vi "logic-train-sample-7-1-ALT.vi"(11 "Request\nCapture":bool) -> (1 "Hand_Close":bool, 3 "Arm_Extend":bool, 4 "State":T1)   [LabVIEW 2020]
uses:
  sample-7-1-state-enum.ctl
  <vilib>/Utility/semaphor.llb/Obtain Semaphore Reference.vi
  <vilib>/Rock Robotics/WPI/ThirdParty/JAS_Junk/TrajLib/Timer_Reset.vi
  <vilib>/Rock Robotics/WPI/ThirdParty/JAS_Junk/TrajLib/Timer_Start.vi
  <vilib>/Rock Robotics/WPI/ThirdParty/JAS_Junk/TrajLib/Timer_Stop.vi
  <vilib>/Rock Robotics/WPI/ThirdParty/JAS_Junk/TrajLib/Trajectory_Library.lvlib
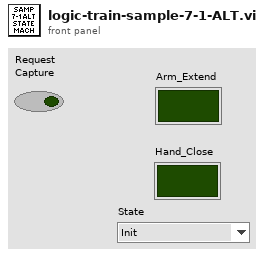
[diagram p1: front panel]
types:
  T1 = typedef "sample-7-1-state-enum.ctl" = enum16{"Init", "ExtendArm", "ExtendArmWait", "CloseHand", "CloseHandWait", "RetractArm", "RetractArmWait", "OpenHand", "OpenHandWait", "Ready"}
  T2 = typedef "Trajectory_Library.lvlib/TIMER.ctl" = cluster{"StartTime":dbl, "Accumulated TIme":dbl, "Running":bool, "semaphore":T3}
  T3 = typedef "Semaphore RefNum" = refnum<k1>
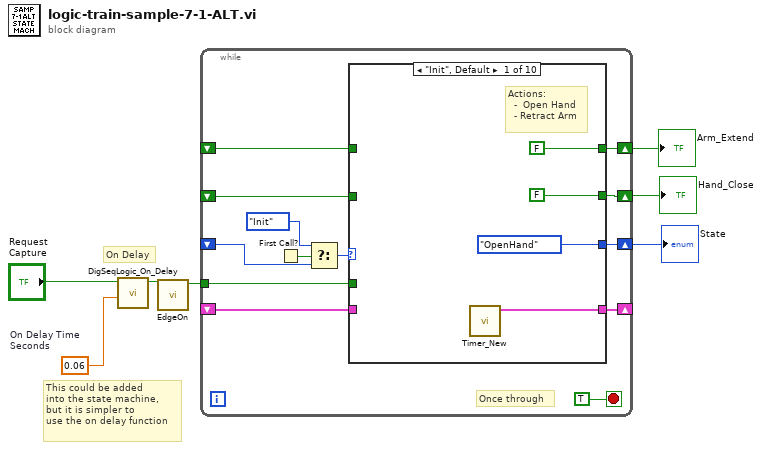
[diagram p0: block diagram]
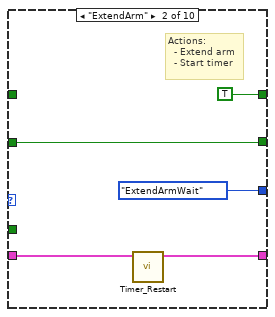
[diagram p2: hidden frame]
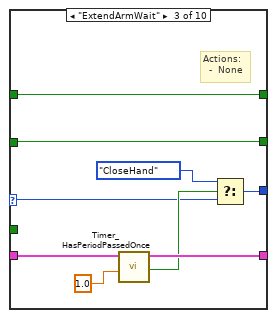
[diagram p3: hidden frame]
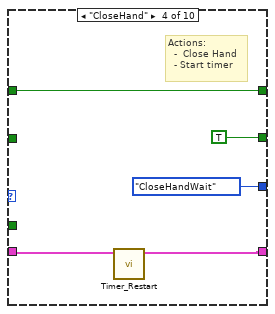
[diagram p4: hidden frame]
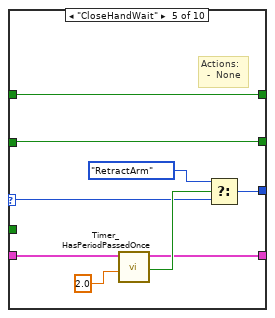
[diagram p5: hidden frame]
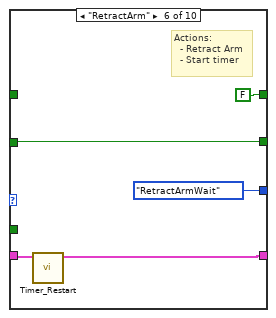
[diagram p6: hidden frame]
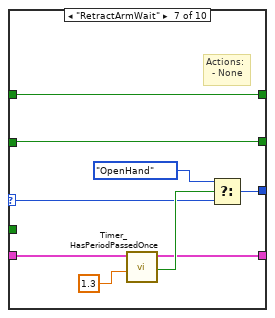
[diagram p7: hidden frame]
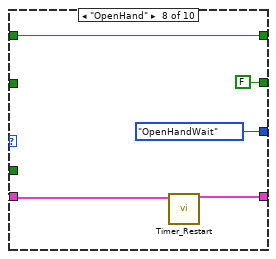
[diagram p8: hidden frame]
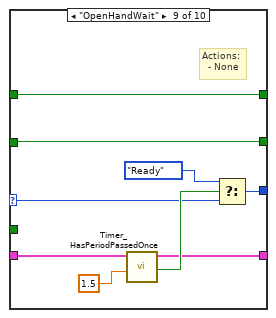
[diagram p9: hidden frame]
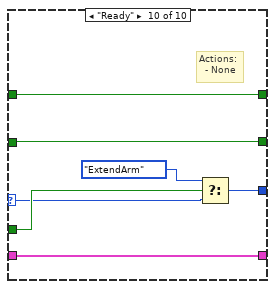
[diagram p10: hidden frame]
diagram:
  w7 = 0.06  # On Delay Time Seconds
  # "This could be added\ninto the state machine,\nbut it is simpler to \nuse the on delay function"
  # "On Delay"
  n1 = call <vilib>:"DigSeqLogic_On_Delay.vi"("Delay"=w7, "Input"="Request\nCapture") -> ("Output"=w6:bool)  [unwired: 8 in, 1 out]
  n2 = call "EdgeOn.vi"("Input"=w6) -> ("Edge On"=w4:bool)  [unwired: 10 in]
  n3 = while {
    shift-right: [w13] -> w1
    shift-left: _ -> [w16]
    shift-right: [w14] -> w2
    shift-left: _ -> [w19]
    shift-right: [w15] -> w3
    shift-left: _ -> [w10]
    shift-right: [w12] -> _
    shift-left: _ -> [w20]
    tunnel: w4 -> [w18]
    stop <- TRUE stop-if-true
    # "Once through"
    n4 = First Call?() -> (First Call?: T/F=w9:bool)
    n5 = Select(t=sample-7-1-state-enum."Init" ("Sample-7-1-State"), s=w9, f=w10) -> (s? t:f=w11:T1)
    n6 = case shown="\"Init\", Default" w11 {
      selector: w11 -> [_ _ w30 _ w48 _ w63 _ w76 w83]
      tunnel: [FALSE TRUE w37 w43 w44 FALSE w59 w68 w72 w87] -> w13
      tunnel: [FALSE w28 w38 TRUE w45 w54 w58 FALSE w73 w86] -> w14
      tunnel: [sample-7-1-state-enum."OpenHand" ("Sample-7-1-State") sample-7-1-state-enum."ExtendArmWait" ("Sample-7-1-State") w32 sample-7-1-state-enum."CloseHandWait" ("Sample-7-1-State") w49 sample-7-1-state-enum."RetractArmWait" ("Sample-7-1-State") w62 sample-7-1-state-enum."OpenHandWait" ("Sample-7-1-State") w77 w81] -> w15
      tunnel: [w21 w25 w35 w42 w46 w57 w60 w70 w74 w85] -> w12
      tunnel: w20 -> [_ w26 w34 w41 w47 w53 w61 w69 w75 w85]
      tunnel: w19 -> [_ w28 w38 _ w45 w54 w58 _ w73 w86]
      tunnel: w16 -> [_ _ w37 w43 w44 _ w59 w68 w72 w87]
      tunnel: w18 -> [_ _ _ _ _ _ _ _ _ w84]
      frame "Init", Default {
        # "Actions:\n  -  Open Hand\n  - Retract Arm"
        n7 = call <vilib>:"Timer_New.vi"() -> ("TIMER"=w21:T2)  [unwired: 11 in]
      }
      frame "ExtendArm" {
        # "Actions:\n  - Extend arm\n  - Start timer"
        n8 = call <vilib>:"Timer_Restart.vi"("in Timer"=w26) -> ("out Timer"=w25:T2)  [unwired: 10 in]
      }
      frame "ExtendArmWait" {
        # "Actions:\n  -  None"
        n9 = call <vilib>:"Timer_HasPeriodPassedOnce.vi"("Period"=1.0, "in Timer"=w34) -> ("Expired"=w31:bool, "out Timer"=w35:T2)  [unwired: 7 in, 1 out]
        n10 = Select(t=sample-7-1-state-enum."CloseHand" ("Sample-7-1-State"), s=w31, f=w30) -> (s? t:f=w32:T1)
      }
      frame "CloseHand" {
        # "Actions:\n  -  Close Hand\n  - Start timer"
        n11 = call <vilib>:"Timer_Restart.vi"("in Timer"=w41) -> ("out Timer"=w42:T2)  [unwired: 10 in]
      }
      frame "CloseHandWait" {
        # "Actions:\n  -  None"
        n12 = call <vilib>:"Timer_HasPeriodPassedOnce.vi"("Period"=2.0, "in Timer"=w47) -> ("Expired"=w50:bool, "out Timer"=w46:T2)  [unwired: 7 in, 1 out]
        n13 = Select(t=sample-7-1-state-enum."RetractArm" ("Sample-7-1-State"), s=w50, f=w48) -> (s? t:f=w49:T1)
      }
      frame "RetractArm" {
        # "Actions:\n  - Retract Arm\n  - Start timer"
        n14 = call <vilib>:"Timer_Restart.vi"("in Timer"=w53) -> ("out Timer"=w57:T2)  [unwired: 10 in]
      }
      frame "RetractArmWait" {
        # "Actions:\n  - None"
        n15 = call <vilib>:"Timer_HasPeriodPassedOnce.vi"("Period"=1.3, "in Timer"=w61) -> ("Expired"=w64:bool, "out Timer"=w60:T2)  [unwired: 7 in, 1 out]
        n16 = Select(t=sample-7-1-state-enum."OpenHand" ("Sample-7-1-State"), s=w64, f=w63) -> (s? t:f=w62:T1)
      }
      frame "OpenHand" {
        n17 = call <vilib>:"Timer_Restart.vi"("in Timer"=w69) -> ("out Timer"=w70:T2)  [unwired: 10 in]
      }
      frame "OpenHandWait" {
        # "Actions:\n  - None"
        n18 = call <vilib>:"Timer_HasPeriodPassedOnce.vi"("Period"=1.5, "in Timer"=w75) -> ("Expired"=w78:bool, "out Timer"=w74:T2)  [unwired: 7 in, 1 out]
        n19 = Select(t=sample-7-1-state-enum."Ready" ("Sample-7-1-State"), s=w78, f=w76) -> (s? t:f=w77:T1)
      }
      frame "Ready" {
        # "Actions:\n  - None"
        n20 = Select(t=sample-7-1-state-enum."ExtendArm", s=w84, f=w83) -> (s? t:f=w81:T1)
      }
    }
  }
  "State" <- w3
  "Arm_Extend" <- w1
  "Hand_Close" <- w2
